vi "Simple_Example.vi"() -> ()   [LabVIEW 2019]
doc: "This example shows a simple recording of an image sequence and the image access afterwards.\nIt is a good starting point for writing own applications.\nBut it will not be fail save, i.e. doesnt react on errors, just handles them forward to the end\n\nUsage:\nSelect your required image count before you start the program.\nOnce started, the camera class will be initialized and images will be recorded automatically.\nWhen acquisition has finished you can address the images and set a certain roi \nTo finish the program click on quit application, this will force fan exit of the camera class"
uses:
  camera/Camera.lvclass
  <vilib>/picture/picture.llb/Draw 8-Bit Pixmap.vi
  <vilib>/picture/picture.llb/Draw True-Color Pixmap.vi
panel:
  out "colormap(U8)":u32[](array[numeric])
  out "Image(U16)":u16[][](graph)
  in  "Zoom [%]":i32(slide)=26 min=10 max=200 step=5 scale=10.0..200.0
  out "Image":picture
  out "rawImage":u16[][](array[numeric])
  in  "data_format":T1(ring)=enum."Mono16"
  in  "Image Index":u32 max=9
  out "Recorded Images":u32
  in  "Quit":bool
  in  "cropY1":u64=2 min=2 max=2048 step=1
  in  "cropX1":u64=2 min=2 max=2048 step=1
  in  "cropY0":u64=1 min=1 max=2047 step=1
  in  "cropX0":u64=1 min=1 max=2047 step=1
  out "Image Height":u16
  out "Image Width":u16
  in  "dwImgCount":u32=10 caption="Required Number of Images" max=4023
  out "Error":errorcluster {"code" format="%x"}
  # "This example shows a simple recording of an image sequence and the image access afterwards.\nIt is a good starting point for writing own applications.\nBut it will not be fail save, i.e. doesnt react on errors, just handles them forward to the end\n\nUsage:\nSelect your required image count before you start the program.\nOnce started, the camera class will be initialized and images will be recorded automatically.\nWhen acquisition has finished you can address the images and crop them to a smaller size.\nTo finish the program click on quit application, this will force fan exit of the camera class"
  # "pco.labview"
  # "Camera Setup"
  # "Recording Control"
  # "Parameters for image readout"
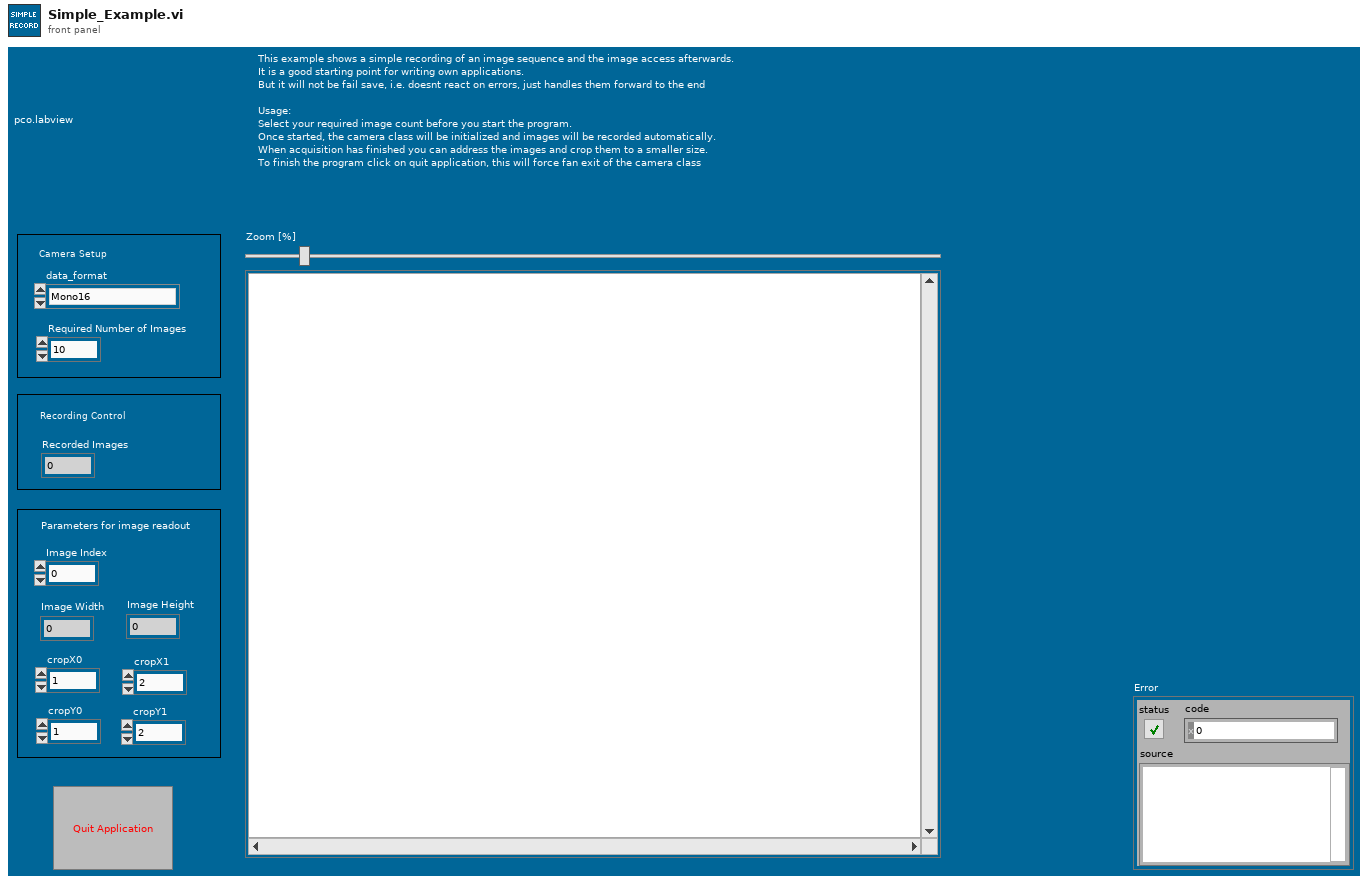
[diagram p1: front panel]
types:
  T1 = enum16{"Undefined", "Mono8", "Mono16", "BGRA8", "RGBA8", "BGRA16", "RGBA16", "CompressedMono8"}
  T2 = enum8{"Enabled", "Disabled", "Disabled and Grayed Out"}
  T3 = enum16{"sequence", "sequence non blocking", "ring buffer", "fifo", "tif", "multitif", "pcoraw", "b16", "dicom", "multidicom", "camram_ring", "camram_segment"}
  T4 = typedef "Camera.lvclass/binning.ctl" = cluster{"vert":u16, "horz":u16, "mode":u16}
  T5 = cluster{"exposure_time_s":dbl, "delay_time_s":dbl, "roi":cluster{"x0":u64, "y0":u64, "x1":u64, "y1":u64}, "timestamp_mode":u16, "pixelrate":u32, "conversion_factor":sgl, "trigger_mode":u16, "acquire_mode":u16, "acquire_sequence_number":u32, "metadata_mode":u16, "noisefilter_mode":u16, "pixel_format":u32, "binning":T4, "auto_exposure":cluster{"region":u16, "min_exposure_s":dbl, "max_exposure_s":dbl}}
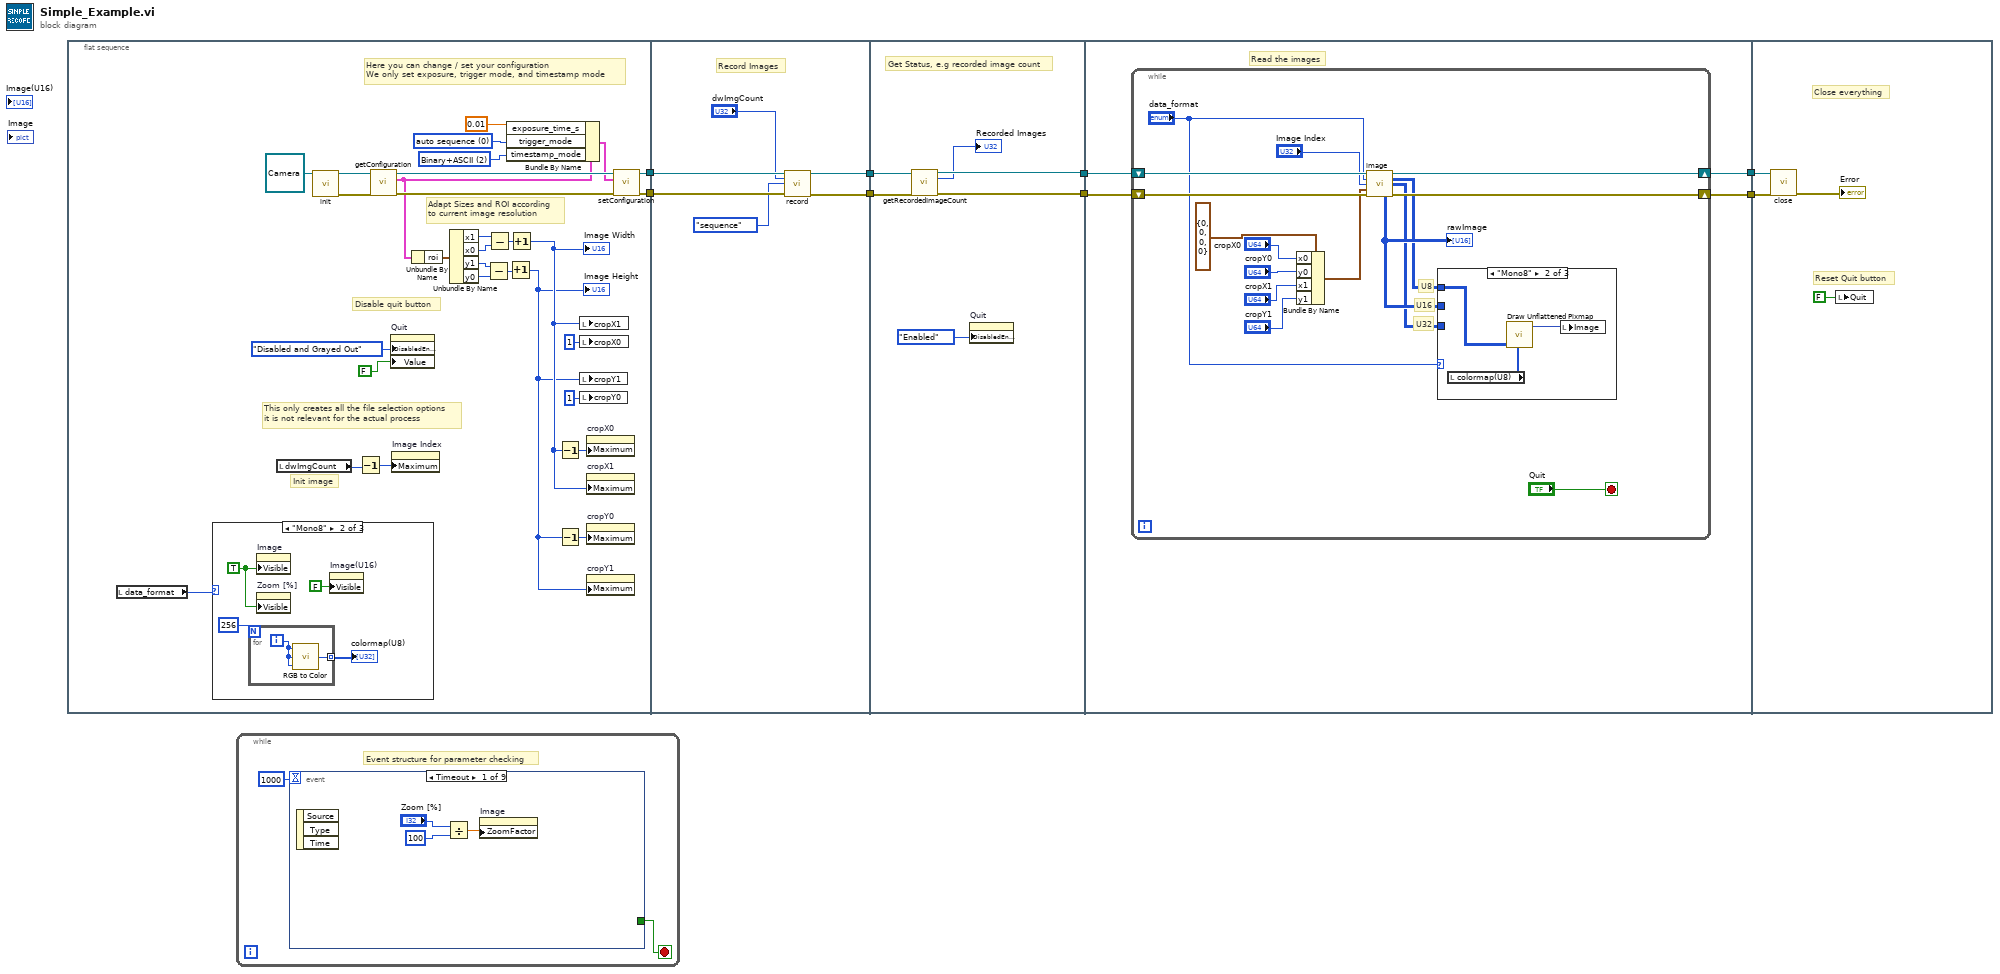
[diagram p0: block diagram]
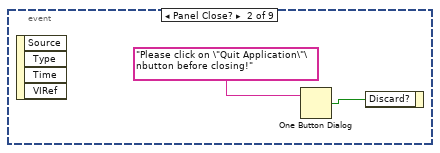
[diagram p2: hidden frame]
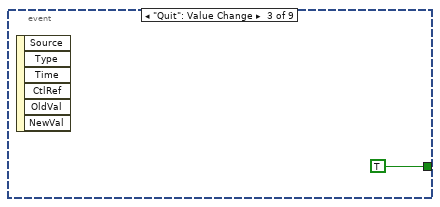
[diagram p3: hidden frame]
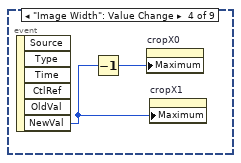
[diagram p4: hidden frame]
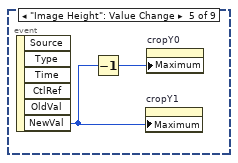
[diagram p5: hidden frame]
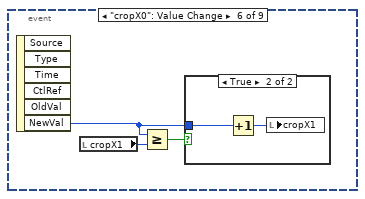
[diagram p6: hidden frame]
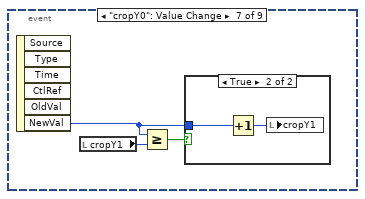
[diagram p8: hidden frame]
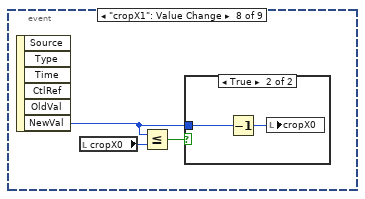
[diagram p10: hidden frame]
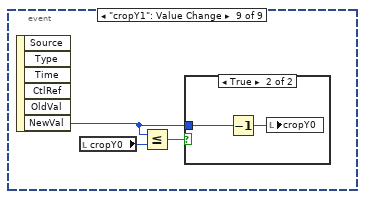
[diagram p12: hidden frame]
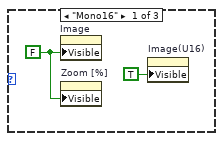
[diagram p14: hidden frame]
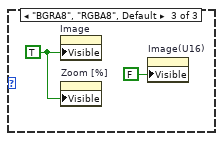
[diagram p15: hidden frame]
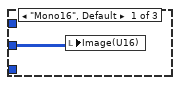
[diagram p16: hidden frame]
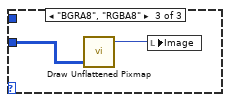
[diagram p17: hidden frame]
diagram:
  n1 = flat-sequence {
    tunnel: [w31] -> w8
    tunnel: [w30] -> w7
    tunnel: w8 -> [w54]
    tunnel: w7 -> [w53]
    tunnel: [w51] -> w6
    tunnel: [w50] -> w5
    tunnel: w6 -> [w60]
    tunnel: w5 -> [w59]
    tunnel: [w58] -> w4
    tunnel: [w57] -> w3
    tunnel: w4 -> [w63]
    tunnel: w3 -> [w64]
    tunnel: [w62] -> w2
    tunnel: [w61] -> w1
    tunnel: w2 -> [w88]
    tunnel: w1 -> [w87]
    frame #0 {
      w15 = u16 2 items=["OFF", "Binary", "Binary+ASCII", "ASCII"] ("TimestampMode")
      w35 = u16 0 items=["auto sequence"=0, "software trigger"=1, "external exposure start & software trigger"=2, "external exposure control"=3, "external synchronized"=4, "fast external exposure control"=5, "external CDS control"=6, "slow external exposure control"=7, "external synchronized HDSDI"=258] ("TriggerMode")
      # "Here you can change / set your configuration\nWe only set exposure, trigger mode, and timestamp mode"
      # "Init image"
      # "This only creates all the file selection options\nit is not relevant for the actual process"
      # "Adapt Sizes and ROI according\nto current image resolution"
      # "Disable quit button"
      n2 = local read "data_format"() -> (w10:T1)
      n3 = case shown="\"Mono8\"" w10 {
        frame "Mono16" {
          w40 = FALSE ("Visible")
          n4 = property on="Image" class="Pict"("Visible"=w40) -> ()  [unwired: 2 in, 2 out]
          n5 = property on="Zoom [%]" class="Slide (strict)"("Visible"=w40) -> ()  [unwired: 2 in, 2 out]
          n6 = property on="Image(U16)" class="IntGraph (strict)"("Visible"=TRUE) -> ()  [unwired: 2 in, 2 out]
        }
        frame "Mono8" {
          w43 = TRUE ("Visible")
          n7 = for {
            N: 256 -> [_]
            tunnel: [w45] -> w42 mode=indexing
            i -> [w46]
            n8 = call <vilib>:"RGB to Color.vi"("B"=w46, "G"=w46, "R"=w46) -> ("Color"=w45:u32)
          }
          "colormap(U8)" <- w42
          n9 = property on="Image" class="Pict"("Visible"=w43) -> ()  [unwired: 2 in, 2 out]
          n10 = property on="Zoom [%]" class="Slide (strict)"("Visible"=w43) -> ()  [unwired: 2 in, 2 out]
          n11 = property on="Image(U16)" class="IntGraph (strict)"("Visible"=FALSE) -> ()  [unwired: 2 in, 2 out]
        }
        frame "BGRA8", "RGBA8", Default {
          w47 = TRUE ("Visible")
          n12 = property on="Image" class="Pict"("Visible"=w47) -> ()  [unwired: 2 in, 2 out]
          n13 = property on="Zoom [%]" class="Slide (strict)"("Visible"=w47) -> ()  [unwired: 2 in, 2 out]
          n14 = property on="Image(U16)" class="IntGraph (strict)"("Visible"=FALSE) -> ()  [unwired: 2 in, 2 out]
        }
      }
      n15 = local read "dwImgCount"() -> (w11:u32)
      n16 = call-dynamic "init.vi"("Camera in"=refnum<class "Camera.lvclass"> refnum ("PCOCamera in")) -> ("Camera out"=w37:refnum<class "Camera.lvclass">, "error out"=w36:errorcluster)  [unwired: 8 in]
      n17 = Decrement(x=w11) -> (x-1=w12:u32)
      n18 = call-dynamic "getConfiguration.vi"("error in (no error)"=w36, "Camera in"=w37) -> ("error out"=w33:errorcluster, "configuration"=w25:T5, "Camera out"=w34:refnum<class "Camera.lvclass">)  [unwired: 7 in]
      n19 = property on="Quit" class="Bool (strict)"("DisabledEnum"=T2."Disabled and Grayed Out" ("Disabled"), "Value"=FALSE ("Stop")) -> ()  [unwired: 2 in, 2 out]
      n20 = property on="Image Index" class="DigNum (strict)"("Maximum"=w12) -> ()  [unwired: 2 in, 2 out]
      n21 = Unbundle By Name(w25) -> ("roi"=w24:cluster{"x0":u64, "y0":u64, "x1":u64, "y1":u64})
      n22 = Unbundle By Name(w24) -> ("x1"=w22:u64, "x0"=w23:u64, "y1"=w20:u64, "y0"=w21:u64)
      n23 = Subtract(x=w20, y=w21) -> (x-y=w18:u64)
      n24 = Subtract(x=w22, y=w23) -> (x-y=w19:u64)
      n25 = Bundle By Name(cluster=w25, "exposure_time_s"=0.01, "trigger_mode"=w35, "timestamp_mode"=w15) -> (w32:T5)
      n26 = Increment(x=w18) -> (x+1=w16:u64)
      "Image Height" <- w16
      n27 = Increment(x=w19) -> (x+1=w17:u64)
      "Image Width" <- w17
      n28 = Decrement(x=w17) -> (x-1=w27:u64)
      n29 = Decrement(x=w16) -> (x-1=w26:u64)
      n30 = local write "cropX1"(w17) -> ()
      n31 = local write "cropX0"(u16 1 ("roiY0")) -> ()
      n32 = local write "cropY1"(w16) -> ()
      n33 = local write "cropY0"(u16 1 ("roiY0")) -> ()
      n34 = property on="cropX0" class="DigNum (strict)"("Maximum"=w27) -> ()  [unwired: 2 in, 2 out]
      n35 = property on="cropX1" class="DigNum (strict)"("Maximum"=w17) -> ()  [unwired: 2 in, 2 out]
      n36 = property on="cropY0" class="DigNum (strict)"("Maximum"=w26) -> ()  [unwired: 2 in, 2 out]
      n37 = property on="cropY1" class="DigNum (strict)"("Maximum"=w16) -> ()  [unwired: 2 in, 2 out]
      n38 = call-dynamic "setConfiguration.vi"("error in (no error)"=w33, "configuration"=w32, "Camera in"=w34) -> ("error out"=w30:errorcluster, "Camera out"=w31:refnum<class "Camera.lvclass">)  [unwired: 7 in]
    }
    frame #1 {
      # "Record Images"
      n39 = call-dynamic "record.vi"("Camera in"=w54, "num_images"="dwImgCount", "record_mode"=T3."sequence", "error in (no error)"=w53) -> ("Camera out"=w51:refnum<class "Camera.lvclass">, "error out"=w50:errorcluster)  [unwired: 10 in]
    }
    frame #2 {
      # "Get Status, e.g recorded image count"
      n40 = call-dynamic "getRecordedImageCount.vi"("Camera in"=w60, "error in (no error)"=w59) -> ("Camera out"=w58:refnum<class "Camera.lvclass">, "recorded_image_count"=→"Recorded Images":u32, "error out"=w57:errorcluster)  [unwired: 11 in]
      n41 = property on="Quit" class="Bool (strict)"("DisabledEnum"=T2."Enabled" ("Disabled")) -> ()  [unwired: 2 in, 2 out]
    }
    frame #3 {
      # "Read the images"
      n42 = while {
        shift-right: [w78] -> w62
        shift-left: w63 -> [w80]
        shift-right: [w73] -> w61
        shift-left: w64 -> [w79]
        stop <- "Quit" stop-if-true
        # "U32"
        # "U16"
        # "U8"
        n43 = Bundle By Name(cluster=cluster{"x0":u64, "y0":u64, "x1":u64, "y1":u64} {"x0"=0, "y0"=0, "x1"=0, "y1"=0} ("roi"), "x0"="cropX0", "y0"="cropY0", "x1"="cropX1", "y1"="cropY1") -> (w72:cluster{"x0":u64, "y0":u64, "x1":u64, "y1":u64})
        n44 = call-dynamic "image.vi"("Camera in"=w80, "data_format"="data_format", "image_index"="Image Index", "crop"=w72, "error in (no error)"=w79) -> ("Camera out"=w78:refnum<class "Camera.lvclass">, "image (U8)"=w65:u8[][], "image (U32)"=w66:u32[][], "raw_image (U16)"=w67:u16[][], "error out"=w73:errorcluster)  [unwired: 2 in, 4 out]
        "rawImage" <- w67
        n45 = case shown="\"Mono8\"" "data_format" {
          tunnel: w66 -> [_ _ w86]
          tunnel: w65 -> [_ w83 _]
          tunnel: w67 -> [w81 _ _]
          frame "Mono16", Default {
            n46 = local write "Image(U16)"(w81) -> ()
          }
          frame "Mono8" {
            n47 = local read "colormap(U8)"() -> (w82:u32[])
            n48 = call-poly <vilib>:"Draw Unflattened Pixmap.vi"("data"=w83, "color table"=w82) -> ("new picture"=w84:picture)  [unwired: 7 in]
            n49 = local write "Image"(w84) -> ()
          }
          frame "BGRA8", "RGBA8" {
            n50 = call-poly <vilib>:"Draw Unflattened Pixmap.vi"("data (RGB format)"=w86) -> ("new picture"=w85:picture)  [unwired: 8 in]
            n51 = local write "Image"(w85) -> ()
          }
        }
      }
    }
    frame #4 {
      # "Reset Quit button"
      # "Close everything"
      n52 = call-dynamic "close.vi"("error in (no error)"=w87, "Camera in"=w88) -> ("error out"=→"Error":errorcluster)  [unwired: 9 in]
      n53 = local write "Quit"(FALSE ("Stop")) -> ()
    }
  }
  n54 = while {
    stop <- w91 stop-if-true
    # "Event structure for parameter checking"
    n55 = event shown="[0] Timeout" {
      selector: _ -> [_ _ _ _ _ _ _ _ _]
      dyn-events: _ -> [_ _ _ _ _ _ _ _ _]
      timeout: 1000 -> [_ _ _ _ _ _ _ _ _]
      tunnel: [_ _ TRUE _ _ _ _ _ _] -> w91
      event Timeout {
        n56 = event-data() -> ()  [unwired: 1 in, 3 out]
        n57 = Divide(x="Zoom [%]", y=100 ("Zoom [%]")) -> (x/y=w93:dbl)
        n58 = property on="Image" class="Pict"("ZoomFactor"=w93) -> ()  [unwired: 2 in, 2 out]
      }
      event Panel Close? {
        n59 = event-data() -> ()  [unwired: 1 in, 4 out]
        n60 = One Button Dialog(message="Please click on \"Quit Application\"\nbutton before closing!") -> (true=w96:bool)  [unwired: 1 in]
        n61 = event-data("Discard?"=w96) -> ()  [unwired: 1 in, 1 out]
      }
      event "Quit": Value Change {
        n62 = event-data() -> ()  [unwired: 1 in, 6 out]
      }
      event "Image Width": Value Change {
        n63 = event-data() -> ("NewVal"=w99:u16)  [unwired: 1 in, 5 out]
        n64 = Decrement(x=w99) -> (x-1=w100:u16)
        n65 = property on="cropX0" class="DigNum (strict)"("Maximum"=w100) -> ()  [unwired: 2 in, 2 out]
        n66 = property on="cropX1" class="DigNum (strict)"("Maximum"=w99) -> ()  [unwired: 2 in, 2 out]
      }
      event "Image Height": Value Change {
        n67 = event-data() -> ("NewVal"=w101:u16)  [unwired: 1 in, 5 out]
        n68 = Decrement(x=w101) -> (x-1=w102:u16)
        n69 = property on="cropY1" class="DigNum (strict)"("Maximum"=w101) -> ()  [unwired: 2 in, 2 out]
        n70 = property on="cropY0" class="DigNum (strict)"("Maximum"=w102) -> ()  [unwired: 2 in, 2 out]
      }
      event "cropX0": Value Change {
        n71 = event-data() -> ("NewVal"=w103:u64)  [unwired: 1 in, 5 out]
        n72 = local read "cropX1"() -> (w105:u64)
        n73 = Greater Or Equal?(x=w103, y=w105) -> (x >= y?=w104:bool)
        n74 = case shown="True" w104 {
          tunnel: w103 -> [_ w107]
          frame False {
          }
          frame True {
            n75 = Increment(x=w107) -> (x+1=w106:u64)
            n76 = local write "cropX1"(w106) -> ()
          }
        }
      }
      event "cropY0": Value Change {
        n77 = event-data() -> ("NewVal"=w108:u64)  [unwired: 1 in, 5 out]
        n78 = local read "cropY1"() -> (w110:u64)
        n79 = Greater Or Equal?(x=w108, y=w110) -> (x >= y?=w109:bool)
        n80 = case shown="True" w109 {
          tunnel: w108 -> [_ w112]
          frame False {
          }
          frame True {
            n81 = Increment(x=w112) -> (x+1=w111:u64)
            n82 = local write "cropY1"(w111) -> ()
          }
        }
      }
      event "cropX1": Value Change {
        n83 = event-data() -> ("NewVal"=w113:u64)  [unwired: 1 in, 5 out]
        n84 = local read "cropX0"() -> (w115:u64)
        n85 = Less Or Equal?(x=w113, y=w115) -> (x <= y?=w114:bool)
        n86 = case shown="True" w114 {
          tunnel: w113 -> [_ w117]
          frame False {
          }
          frame True {
            n87 = Decrement(x=w117) -> (x-1=w116:u64)
            n88 = local write "cropX0"(w116) -> ()
          }
        }
      }
      event "cropY1": Value Change {
        n89 = event-data() -> ("NewVal"=w118:u64)  [unwired: 1 in, 5 out]
        n90 = local read "cropY0"() -> (w120:u64)
        n91 = Less Or Equal?(x=w118, y=w120) -> (x <= y?=w119:bool)
        n92 = case shown="True" w119 {
          tunnel: w118 -> [_ w122]
          frame False {
          }
          frame True {
            n93 = Decrement(x=w122) -> (x-1=w121:u64)
            n94 = local write "cropY0"(w121) -> ()
          }
        }
      }
    }
  }
